vi "Standard Deviation PtByPt.vi"(0 "x":dbl format="%0.2f", 1 "sample length":i32=100, 2 "initialize":bool) -> (3 "standard deviation":dbl format="%0.2f", 4 "mean":dbl format="%0.2f", 5 "error":i32)   [LabVIEW 2020, in "NI_PtbyPt.lvlib"]
doc: "Computes the <B>mean</B> and the <B>standard deviation</B> of the values in the set of input data points specified by <B>sample length</B>."
uses:
  NI_PtbyPt.lvlib
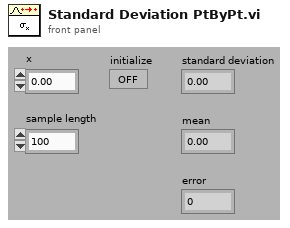
[diagram p1: front panel]
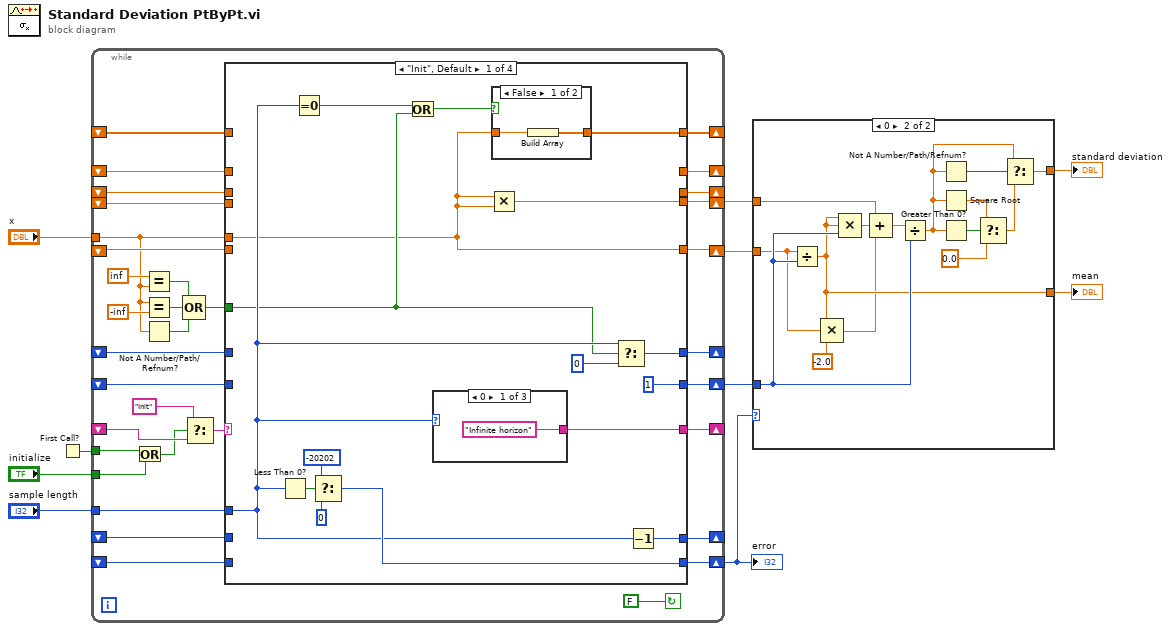
[diagram p0: block diagram]
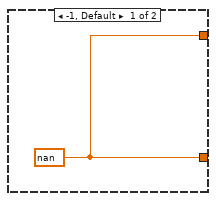
[diagram p2: hidden frame]
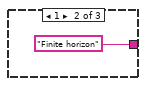
[diagram p4: hidden frame]
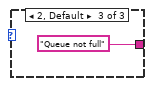
[diagram p5: hidden frame]
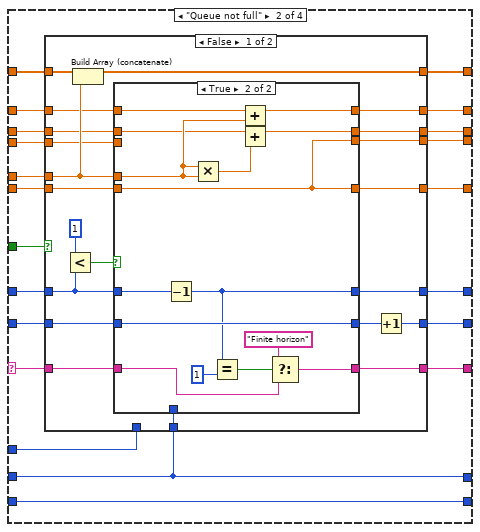
[diagram p6: hidden frame]
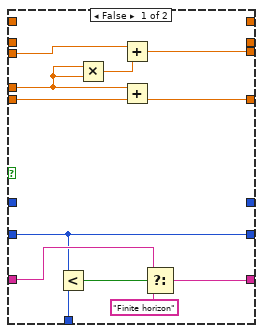
[diagram p7: hidden frame]
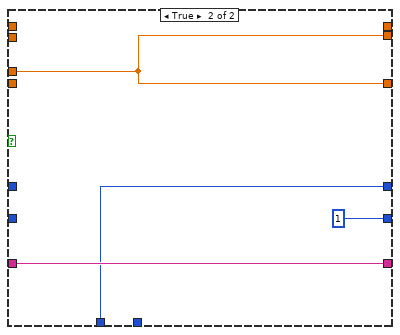
[diagram p8: hidden frame]
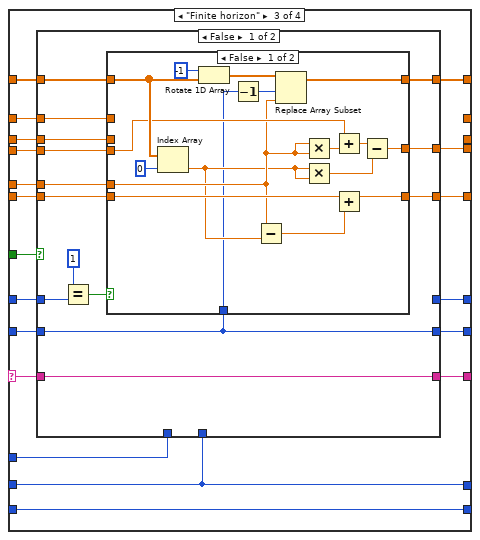
[diagram p9: hidden frame]
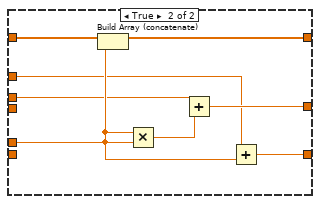
[diagram p10: hidden frame]
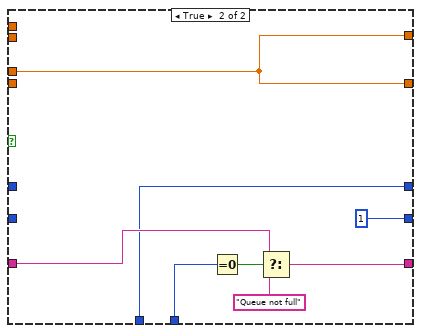
[diagram p11: hidden frame]
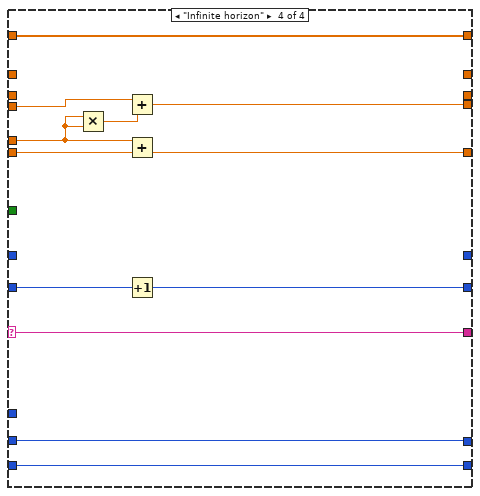
[diagram p12: hidden frame]
diagram:
  n1 = First Call?() -> (First Call?: T/F=w8:bool)
  n2 = while {
    tunnel: w8 -> [w29]
    shift-left: _ -> [w31]
    shift-right: [w32] -> _
    shift-left: _ -> [w33]
    shift-right: [w34] -> w10
    shift-left: _ -> [w36]
    shift-right: [w35] -> _
    shift-left: _ -> [w38]
    shift-right: [w39] -> w9
    shift-left: _ -> [w40]
    shift-right: [w41] -> w6
    shift-left: _ -> [w44]
    shift-right: [w37] -> _
    shift-right: [w22] -> _
    shift-left: _ -> [w21]
    shift-right: [w20] -> _
    shift-left: _ -> [w18]
    shift-right: [w19] -> _
    shift-left: _ -> [w17]
    shift-right: [w15] -> w4
    shift-left: _ -> [w14]
    tunnel: "x" -> [w13]
    tunnel: "sample length" -> [w12]
    tunnel: "initialize" -> [w11]
    stop <- FALSE continue-if-true
    n3 = Or(x=w29, y=w11) -> (x .or. y?=w28:bool)
    n4 = Equal?(x=inf, y=w13) -> (x = y?=w24:bool)
    n5 = Equal?(x=w13, y=-inf) -> (x = y?=w25:bool)
    n6 = Not A Number/Path/Refnum?(number/path/refnum=w13) -> (NaN/Path/Refnum?=w23:bool)
    n7 = Compound Arithmetic op=OR(w24, w25, w23) -> (w16:bool)
    n8 = Select(t="Init", s=w28, f=w44) -> (s? t:f=w42:string)
    n9 = case shown="\"Init\", Default" w42 {
      selector: w42 -> [_ w82 w149 w213]
      tunnel: [w46 w84 w154 w215] -> w41
      tunnel: w40 -> [_ w78 w151 w216]
      tunnel: w13 -> [w46 w80 w150 w211]
      tunnel: [1 w75 w147 w205] -> w39
      tunnel: w38 -> [_ w83 w157 w214]
      tunnel: [w50 w81 w148 w213] -> w37
      tunnel: w36 -> [_ w86 w155 w212]
      tunnel: [w45 w85 w156 w212] -> w35
      tunnel: w12 -> [w51 w67 w140 _]
      tunnel: [w56 w79 w152 w210] -> w34
      tunnel: w33 -> [_ w77 w153 w207]
      tunnel: [w54 w76 w146 w209] -> w32
      tunnel: w31 -> [_ w76 w146 w209]
      tunnel: w16 -> [w48 w74 w144 _]
      tunnel: [w55 w68 w145 _] -> w22
      tunnel: w21 -> [_ w69 w141 _]
      tunnel: [_ w73 _ _] -> w20
      tunnel: [_ w72 _ _] -> w19
      tunnel: w18 -> [_ w71 w143 _]
      tunnel: w17 -> [_ w70 w142 _]
      tunnel: [w52 w66 w139 w206] -> w15
      tunnel: w14 -> [_ w66 w139 w206]
      frame "Init", Default {
        n10 = Less Than 0?(x=w51) -> (x < 0?=w57:bool)
        n11 = Equal To 0?(x=w51) -> (x = 0?=w49:bool)
        n12 = Select(t=-20202, s=w57, f=0) -> (s? t:f=w52:i32)
        n13 = Or(x=w49, y=w48) -> (x .or. y?=w47:bool)
        n14 = case shown="0" w51 {
          tunnel: ["Infinite horizon" "Finite horizon" "Queue not full" ("f")] -> w50
          frame 0 {
          }
          frame 1 {
          }
          frame 2, Default {
          }
        }
        n15 = Multiply(x=w46, y=w46) -> (x*y=w56:dbl)
        n16 = case shown="False" w47 {
          tunnel: w46 -> [w61 _]
          tunnel: [w62 _] -> w45
          frame False {
            n17 = Build Array(w61) -> (w62:dbl[])
          }
          frame True {
          }
        }
        n18 = Select(t=w51, s=w48, f=0) -> (s? t:f=w55:i32)
        n19 = Decrement(x=w51) -> (x-1=w54:i32)
      }
      frame "Queue not full" {
        n20 = case shown="False" w74 {
          tunnel: w86 -> [w107 _]
          tunnel: [w106 _] -> w85
          tunnel: [w105 w137] -> w84
          tunnel: w83 -> [w91 _]
          tunnel: w82 -> [w104 w136]
          tunnel: [w103 w136] -> w81
          tunnel: w80 -> [w102 w137]
          tunnel: [w101 w137] -> w79
          tunnel: w78 -> [w100 _]
          tunnel: w77 -> [w99 _]
          tunnel: w76 -> [w98 _]
          tunnel: [w97 1] -> w75
          tunnel: [w95 _] -> w73
          tunnel: [w94 _] -> w72
          tunnel: w71 -> [w93 _]
          tunnel: w70 -> [w92 _]
          tunnel: w69 -> [w88 _]
          tunnel: [w90 w135] -> w68
          tunnel: w67 -> [_ w135]
          frame False {
            n21 = Less?(x=1, y=w88) -> (x < y?=w89:bool)
            n22 = Build Array (concatenate)(w107, w102) -> (w106:dbl[])
            n23 = case shown="True" w89 {
              tunnel: [w119 w133] -> w105
              tunnel: w91 -> [w108 w124]
              tunnel: w104 -> [w117 w122]
              tunnel: [w115 w123] -> w103
              tunnel: w102 -> [w114 w132]
              tunnel: [w113 w133] -> w101
              tunnel: w100 -> [w112 w133]
              tunnel: w99 -> [w111 _]
              tunnel: w98 -> [w109 _]
              tunnel: [w108 w124] -> w96
              tunnel: [_ w131] -> w95
              tunnel: [_ w130] -> w94
              tunnel: w93 -> [_ w129]
              tunnel: w92 -> [_ w128]
              tunnel: w88 -> [_ w125]
              tunnel: [_ w121] -> w90
              frame False {
                n24 = Less?(x=w108, y=w109) -> (x < y?=w118:bool)
                n25 = Multiply(x=w114, y=w114) -> (x*y=w110:dbl)
                n26 = Add(x=w111, y=w110) -> (x+y=w113:dbl)
                n27 = Add(x=w114, y=w112) -> (x+y=w119:dbl)
                n28 = Select(t=w117, s=w118, f="Finite horizon") -> (s? t:f=w115:string)
              }
              frame True {
                n29 = Decrement(x=w125) -> (x-1=w121:i32)
                n30 = Multiply(x=w132, y=w132) -> (x*y=w134:dbl)
                n31 = Equal?(x=w121, y=1) -> (x = y?=w127:bool)
                n32 = Add(x=w128, y=w132) -> (x+y=w130:dbl)
                n33 = Add(x=w129, y=w134) -> (x+y=w131:dbl)
                n34 = Select(t="Finite horizon" ("f"), s=w127, f=w122) -> (s? t:f=w123:string)
              }
            }
            n35 = Increment(x=w96) -> (x+1=w97:i32)
          }
          frame True {
          }
        }
      }
      frame "Finite horizon" {
        n36 = case shown="False" w144 {
          tunnel: w157 -> [w164 _]
          tunnel: [w171 _] -> w156
          tunnel: w155 -> [w170 _]
          tunnel: [w169 w204] -> w154
          tunnel: w153 -> [w168 _]
          tunnel: [w167 w204] -> w152
          tunnel: w151 -> [w163 _]
          tunnel: w150 -> [w166 w204]
          tunnel: w149 -> [w165 w199]
          tunnel: [w165 w200] -> w148
          tunnel: [w164 1] -> w147
          tunnel: w146 -> [_ w198]
          tunnel: [_ w197] -> w145
          tunnel: w143 -> [w162 _]
          tunnel: w142 -> [w161 _]
          tunnel: w141 -> [w160 _]
          tunnel: w140 -> [_ w197]
          frame False {
            n37 = Equal?(x=1, y=w160) -> (x = y?=w158:bool)
            n38 = case shown="False" w158 {
              tunnel: [w184 w195] -> w171
              tunnel: w170 -> [w183 w196]
              tunnel: [w182 w194] -> w169
              tunnel: w168 -> [w181 _]
              tunnel: [w177 w191] -> w167
              tunnel: w163 -> [w176 _]
              tunnel: w166 -> [w175 w193]
              tunnel: w164 -> [w172 _]
              tunnel: w162 -> [_ w190]
              tunnel: w161 -> [_ w189]
              frame False {
                n39 = Index Array(array=w183, index=0 ("Index")) -> (element=w174:dbl)
                n40 = Rotate 1D Array(1:w183, 2:i16 -1 ("n")) -> (0:w186:dbl[])
                n41 = Decrement(x=w172) -> (x-1=w185:i32)
                n42 = Subtract(x=w175, y=w174) -> (x-y=w173:dbl)
                n43 = Replace Array Subset(array=w186, new element=w175, index=w185) -> (w184:dbl[])
                n44 = Multiply(x=w175, y=w175) -> (x*y=w180:dbl)
                n45 = Multiply(x=w174, y=w174) -> (x*y=w178:dbl)
                n46 = Add(x=w181, y=w180) -> (x+y=w179:dbl)
                n47 = Add(x=w176, y=w173) -> (x+y=w182:dbl)
                n48 = Subtract(x=w179, y=w178) -> (x-y=w177:dbl)
              }
              frame True {
                n49 = Build Array (concatenate)(w196, w193) -> (w195:dbl[])
                n50 = Multiply(x=w193, y=w193) -> (x*y=w192:dbl)
                n51 = Add(x=w190, y=w192) -> (x+y=w191:dbl)
                n52 = Add(x=w189, y=w193) -> (x+y=w194:dbl)
              }
            }
          }
          frame True {
            n53 = Equal To 0?(x=w198) -> (x = 0?=w203:bool)
            n54 = Select(t=w199, s=w203, f="Queue not full") -> (s? t:f=w200:string)
          }
        }
      }
      frame "Infinite horizon" {
        n55 = Multiply(x=w211, y=w211) -> (x*y=w208:dbl)
        n56 = Add(x=w207, y=w208) -> (x+y=w210:dbl)
        n57 = Add(x=w211, y=w216) -> (x+y=w215:dbl)
        n58 = Increment(x=w214) -> (x+1=w205:i32)
      }
    }
  }
  "error" <- w4
  n59 = case shown="0" w4 {
    tunnel: w10 -> [_ w232]
    tunnel: w9 -> [_ w231]
    tunnel: [w217 w230] -> w7
    tunnel: w6 -> [_ w229]
    tunnel: [w217 w219] -> w5
    frame -1, Default {
      w217 = nan
    }
    frame 0 {
      n60 = Divide(x=w229, y=w231) -> (x/y=w230:dbl)
      n61 = Compound Arithmetic op=MULTIPLY(w230, w229, -2.0) -> (w218:dbl)
      n62 = Compound Arithmetic op=MULTIPLY(w230, w230, w231) -> (w227:dbl)
      n63 = Compound Arithmetic op=ADD(w232, w227, w218) -> (w226:dbl)
      n64 = Divide(x=w226, y=w231) -> (x/y=w221:dbl)
      n65 = Not A Number/Path/Refnum?(number/path/refnum=w221) -> (NaN/Path/Refnum?=w222:bool)
      n66 = Square Root(x=w221) -> (sqrt(x)=w224:dbl)
      n67 = Greater Than 0?(x=w221) -> (x > 0?=w225:bool)
      n68 = Select(t=w224, s=w225, f=0.0) -> (s? t:f=w220:dbl)
      n69 = Select(t=w221, s=w222, f=w220) -> (s? t:f=w219:dbl)
    }
  }
  "standard deviation" <- w5
  "mean" <- w7
